vi "Theremin Gain.vi"(5 "Min Amp":dbl, 7 "Max Amp":dbl, 10 "Input Amp":dbl) -> (2 "Output Gain":dbl)   [LabVIEW 2012]
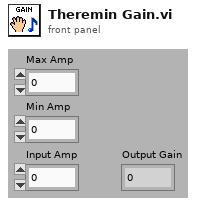
[diagram p1: front panel]
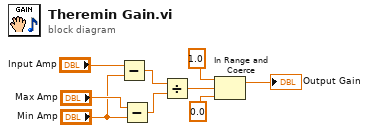
[diagram p0: block diagram]
diagram:
  n1 = Subtract(x="Input Amp", y="Min Amp") -> (x-y=w6:dbl)
  n2 = Subtract(x="Max Amp", y="Min Amp") -> (x-y=w5:dbl)
  n3 = Divide(x=w6, y=w5) -> (x/y=w4:dbl)
  n4 = In Range and Coerce(upper limit=1.0, x=w4, lower limit=0.0) -> (coerced(x)=→"Output Gain":dbl)  [unwired: 1 out]
